vi "ClusterValueChange.vi"(0 "VI Reference":refnum<vi>, 5 "Array":string[](array[string]), 7 "Control Value":variant, 11 "error in":errorcluster) -> (4 "VI Reference out":refnum<vi>, 15 "error out":errorcluster)   [LabVIEW 2016]
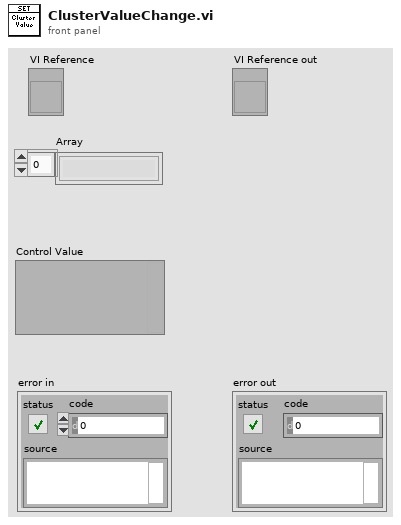
[diagram p1: front panel]
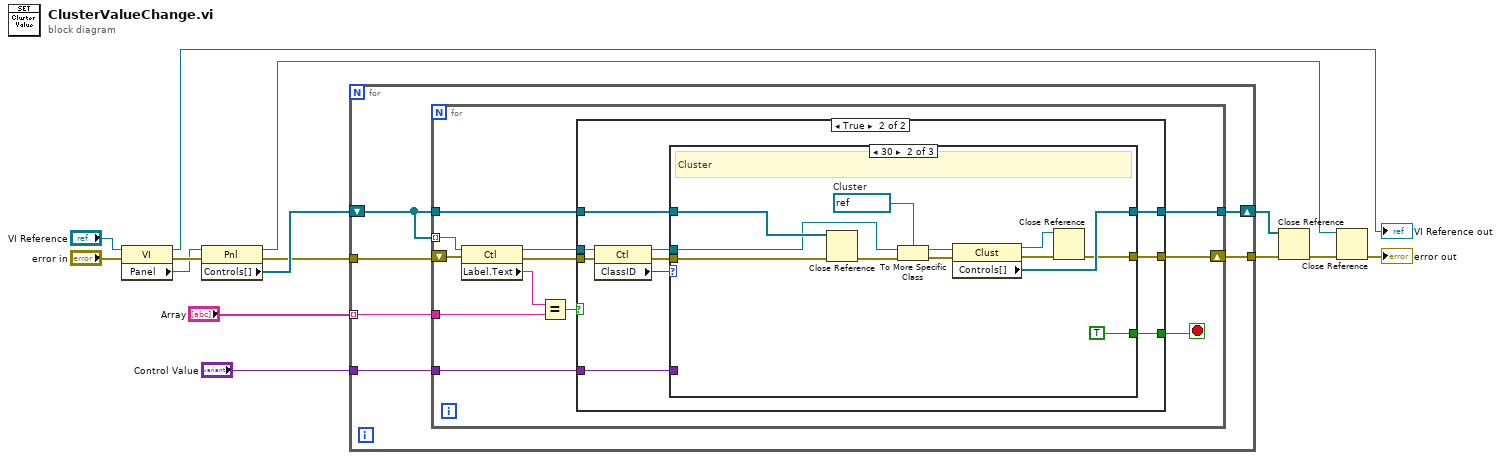
[diagram p0: block diagram]
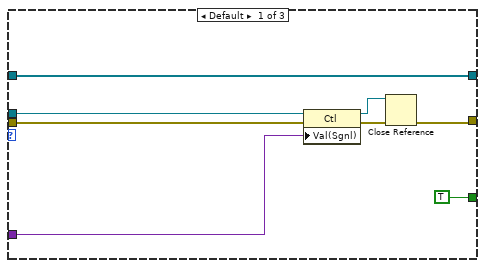
[diagram p3: hidden frame]
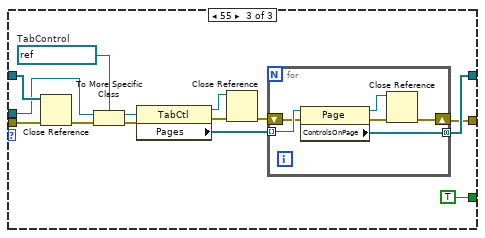
[diagram p4: hidden frame]
diagram:
  n1 = property class="VI"(reference="VI Reference", error in="error in") -> (reference out=→"VI Reference out":refnum<vi>, error out=w14:errorcluster, "Panel"=w13:refnum<vi>)
  n2 = property class="Pnl"(reference=w13, error in=w14) -> (reference out=w2:refnum<vi>, error out=w7:errorcluster, "Controls[]"=w10:refnum<vi>[])
  n3 = for {
    tunnel: "Array" -> [w15] mode=indexing
    tunnel: "Control Value" -> [w20]
    shift-right: [w19] -> w3
    shift-left: w10 -> [w18]
    tunnel: w7 -> [w16]
    tunnel: [w17] -> w5
    n4 = for {
      tunnel: w18 -> [w32] mode=indexing
      tunnel: w15 -> [w21]
      tunnel: w20 -> [w28]
      tunnel: [w26] -> w19
      tunnel: w18 -> [w27]
      shift-right: [w24] -> w17
      shift-left: w16 -> [w23]
      stop <- w22 stop-if-true
      n5 = property class="Ctl"(reference=w32, error in=w23) -> (reference out=w29:refnum<vi>, error out=w25:errorcluster, "Label.Text"=w31:string)
      n6 = Equal?(x=w31, y=w21) -> (x = y?=w30:bool)
      n7 = case shown="True" w30 {
        tunnel: w29 -> [_ w44]
        tunnel: w28 -> [_ w41]
        tunnel: [w33 w40] -> w26
        tunnel: w27 -> [w33 w39]
        tunnel: w25 -> [w34 w37]
        tunnel: [w34 w36] -> w24
        tunnel: [_ w35] -> w22
        frame False {
        }
        frame True {
          n8 = property class="Ctl"(reference=w44, error in=w37) -> (reference out=w42:refnum<vi>, error out=w38:errorcluster, "ClassID"=w43:u32)
          n9 = case shown="30" w43 {
            tunnel: w42 -> [w52 w54 w69]
            tunnel: w41 -> [w51 _ _]
            tunnel: [w50 w63 w74] -> w40
            tunnel: w39 -> [w50 w59 w72]
            tunnel: [TRUE TRUE TRUE] -> w35
            tunnel: w38 -> [w49 w56 w71]
            tunnel: [w47 w57 w73] -> w36
            frame Default {
              n10 = property class="Ctl"(reference=w52, error in=w49, "Val(Sgnl)"=w51) -> (reference out=w46:refnum<vi>, error out=w48:errorcluster)
              n11 = Close Reference(reference=w46, error in (no error)=w48) -> (error out=w47:errorcluster)
            }
            frame 30 {
              w64 = refnum<vi> refnum  # Cluster
              # "Cluster"
              n12 = Close Reference(reference=w59, error in (no error)=w56) -> (error out=w55:errorcluster)
              n13 = To More Specific Class(target class=w64, reference=w54, error in=w55) -> (specific class reference=w62:refnum<vi>, error out=w61:errorcluster)
              n14 = property class="Clust"(reference=w62, error in=w61) -> (reference out=w60:refnum<vi>, error out=w58:errorcluster, "Controls[]"=w63:refnum<vi>[])
              n15 = Close Reference(reference=w60, error in (no error)=w58) -> (error out=w57:errorcluster)
            }
            frame 55 {
              w78 = refnum<vi> refnum  # TabControl
              n16 = Close Reference(reference=w72, error in (no error)=w71) -> (error out=w70:errorcluster)
              n17 = To More Specific Class(target class=w78, reference=w69, error in=w70) -> (specific class reference=w77:refnum<vi>, error out=w76:errorcluster)
              n18 = property class="TabCtl"(reference=w77, error in=w76) -> (reference out=w68:refnum<vi>, error out=w67:errorcluster, "Pages"=w75:refnum<vi>[])
              n19 = Close Reference(reference=w68, error in (no error)=w67) -> (error out=w66:errorcluster)
              n20 = for {
                tunnel: w75 -> [w84] mode=indexing
                tunnel: [w83] -> w74 mode=concatenating
                shift-right: [w80] -> w73
                shift-left: w66 -> [w82]
                n21 = property class="Page"(reference=w84, error in=w82) -> (reference out=w79:refnum<vi>, error out=w81:errorcluster, "ControlsOnPage"=w83:refnum<vi>[])
                n22 = Close Reference(reference=w79, error in (no error)=w81) -> (error out=w80:errorcluster)
              }
            }
          }
        }
      }
    }
  }
  n23 = Close Reference(reference=w3, error in (no error)=w5) -> (error out=w1:errorcluster)
  n24 = Close Reference(reference=w2, error in (no error)=w1) -> (error out=→"error out":errorcluster)
